vi "SetChannelEnable.vi"(7 "LabVIEW Web Service Request":refnum<class "Web Request.lvclass">) -> ()   [LabVIEW 2018]
uses:
  <vilib>/wsapi/Web Request.lvclass
  subvis/Channel Properties.ctl
  CAEN globals.vi
panel:
  in  "Value (Signaling)":T1=enum."Enable"
  in  "error in (no error)":errorcluster
  # "Use the Web Service Request input terminal to call the VIs on the Web Services palette. Do not remove it from the connector pane unless you don't need access to the palette."
  # "Each additional control wired to the connector pane will be available as an input in the URL. To include an indicator in terminal-mode output (the default setting), it must also be wired to the connector pane."
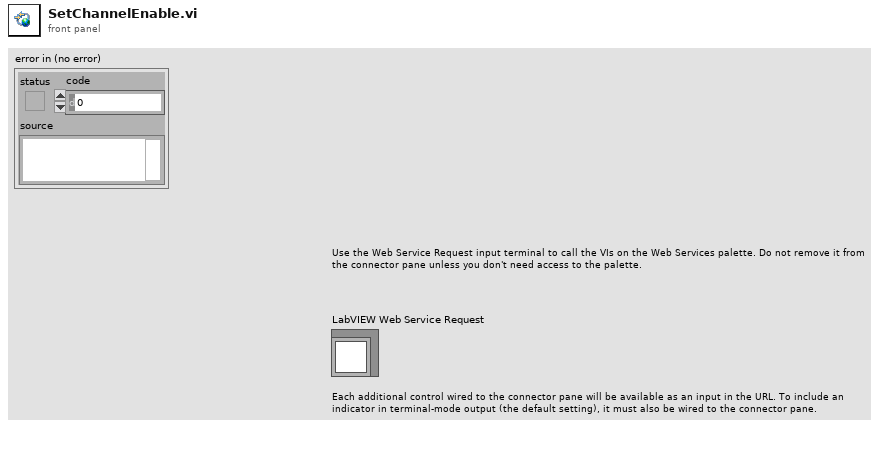
[diagram p1: front panel]
types:
  T1 = typedef "Channel Properties.ctl" = enum16{"Name", "Vset", "Vfile", "Vswmax", "Iset", "Enable", "Flag", "Vbackup"}
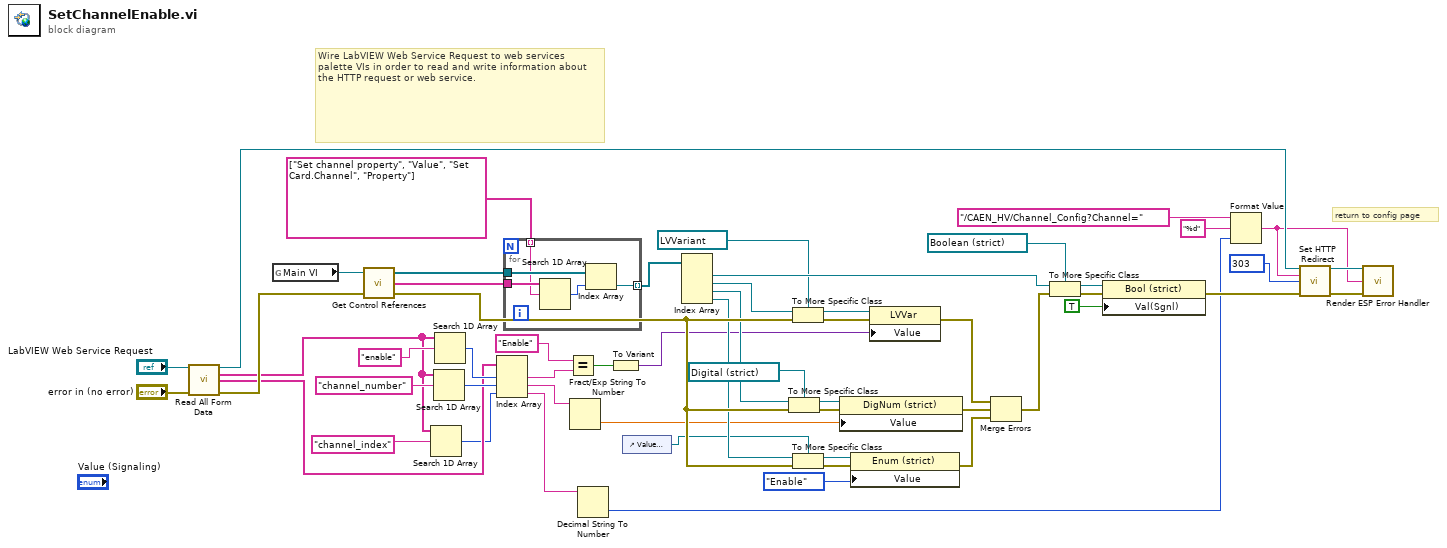
[diagram p0: block diagram]
diagram:
  w50 = 303 items=["100"=100, "101"=101, "200"=200, "201"=201, "202"=202, "203"=203, "204"=204, "205"=205, "206"=206, "300"=300, "301"=301, "302"=302, "303"=303, "304"=304, "305"=305, "306"=306, "307"=307, "400"=400, "401"=401, "402"=402, "403"=403, "404"=404, "405"=405, "406"=406, "407"=407, "408"=408, "409"=409, "410"=410, "411"=411, "412"=412, "413"=413, "414"=414, "415"=415, "416"=416, "417"=417, "500"=500, "501"=501, "502"=502, "503"=503, "504"=504, "505"=505] ("response code (307)")
  # "return to config page"
  # "Wire LabVIEW Web Service Request to web services palette VIs in order to read and write information about the HTTP request or web service."
  n1 = call <vilib>:"Read All Form Data.vi"("LabVIEW Web Service Request"="LabVIEW Web Service Request", "error in (no error)"="error in (no error)") -> ("LabVIEW Web Service Request out"=w26:refnum<class "Web Request.lvclass">, "Key"=w6:string[], "Value"=w7:string[], "error out"=w27:errorcluster)  [unwired: 9 in, 1 out]
  n2 = global read "CAEN globals.vi" "Main VI"() -> (w55:refnum<vi>)
  n3 = call "Get Control References.vi"("error in"=w27, "This vi"=w55) -> ("error out"=w29:errorcluster, "Control Names"=w54:string[], "Controls[]"=w53:refnum<vi>[])  [unwired: 1 in]
  n4 = Search 1D Array(1D array=w6, element="channel_index") -> (index of element=w5:i32)  [unwired: 1 in]
  n5 = Search 1D Array(1D array=w6, element="channel_number") -> (index of element=w45:i32)  [unwired: 1 in]
  n6 = Search 1D Array(1D array=w6, element="enable") -> (index of element=w46:i32)  [unwired: 1 in]
  n7 = Index Array(array=w7, index #1=w46, index #2=w45, index #3=w5) -> (element #1=w15:string, element #2=w17:string, element #3=w4:string)
  n8 = for {
    tunnel: w54 -> [w60]
    tunnel: w53 -> [w59]
    tunnel: [w57] -> w24 mode=indexing
    tunnel: string[] ["Set channel property", "Value", "Set Card.Channel", "Property"] ("Control Names") -> [w56] mode=indexing
    n9 = Search 1D Array(1D array=w60, element=w56) -> (index of element=w58:i32)  [unwired: 1 in]
    n10 = Index Array(array=w59, index=w58) -> (element=w57:refnum<vi>)
  }
  n11 = Equal?(x="Enable", y=w15) -> (x = y?=w14:bool)
  n12 = Fract/Exp String To Number(string=w17) -> (number=w3:dbl)  [unwired: 3 in, 1 out]
  n13 = Decimal String To Number(string=w4) -> (number=w2:i32)  [unwired: 2 in, 1 out]
  n14 = To Variant(anything=w14) -> (Variant=w18:variant)
  n15 = control-ref of="Value (Signaling)"() -> (w1:refnum<vi>)
  n16 = Index Array(array=w24) -> (element #1=w23:refnum<vi>, element #2=w22:refnum<vi>, element #3=w21:refnum<vi>, element #4=w20:refnum<vi>)  [unwired: 4 in]
  n17 = To More Specific Class(target class=refnum<vi> refnum ("number"), reference=w21, error in=w29) -> (specific class reference=w42:refnum<vi>, error out=w41:errorcluster)
  n18 = To More Specific Class(target class=refnum<vi> refnum ("Value"), reference=w22, error in=w29) -> (specific class reference=w51:refnum<vi>, error out=w52:errorcluster)
  n19 = To More Specific Class(target class=w1, reference=w20, error in=w29) -> (specific class reference=w39:refnum<vi>, error out=w40:errorcluster)
  n20 = property class="DigNum (strict)"(reference=w42, error in=w41, "Value"=w3) -> (error out=w32:errorcluster)  [unwired: 1 out]
  n21 = property class="Enum (strict)"(reference=w39, error in=w40, "Value"=Channel_Properties."Enable" ("Value (Signaling)")) -> (error out=w33:errorcluster)  [unwired: 1 out]
  n22 = property class="LVVar"(reference=w51, error in=w52, "Value"=w18) -> (error out=w31:errorcluster)  [unwired: 1 out]
  n23 = Merge Errors(w31, w32, w33) -> (w30:errorcluster)
  n24 = To More Specific Class(target class=refnum<vi> refnum ("replace all? (F)"), reference=w23, error in=w30) -> (specific class reference=w37:refnum<vi>, error out=w36:errorcluster)
  n25 = property class="Bool (strict)"(reference=w37, error in=w36, "Val(Sgnl)"=TRUE ("Value (Signaling)")) -> (error out=w34:errorcluster)  [unwired: 1 out]
  n26 = Format Value(string ("")="/CAEN_HV/Channel_Config?Channel=" ("redirect URL"), format string="%d", value (0)=w2) -> (output string=w10:string)
  n27 = call <vilib>:"Set HTTP Redirect.vi"("LabVIEW Web Service Request"=w26, "redirect URL"=w10, "response code (307)"=w50, "error in (no error)"=w34) -> ("LabVIEW Web Service Request out"=w48:refnum<class "Web Request.lvclass">, "error out"=w49:errorcluster)  [unwired: 10 in]
  n28 = call "Render ESP Error Handler.vi"("LabVIEW Web Service Request"=w48, "Link"=w10, "error in (no error)"=w49) -> ()  [unwired: 11 in, 2 out]
